vi "Rectangle1005.vi"   [LabVIEW 2013]
uses:
  <vilib>/Heliosphere Research LLC/Advanced Plotting Toolkit/api_core/NewPlotProperties.ctl
  <vilib>/Heliosphere Research LLC/Advanced Plotting Toolkit/typedefs/PlotColor.ctl
  <vilib>/Heliosphere Research LLC/Advanced Plotting Toolkit/api_annotations/ShapeProperties.ctl
  <vilib>/Heliosphere Research LLC/Advanced Plotting Toolkit/properties/Line.ctl
  <vilib>/Heliosphere Research LLC/Advanced Plotting Toolkit/properties/Line_Style.ctl
  <vilib>/Heliosphere Research LLC/Advanced Plotting Toolkit/properties/Display.ctl
  <vilib>/Heliosphere Research LLC/Advanced Plotting Toolkit/Advanced Plotting Toolkit.lvlib
types:
  T1 = typedef "Advanced Plotting Toolkit.lvlib/ShapeProperties.ctl" = cluster{"Color":T2, "Line":T3, "Display":T5}
  T2 = typedef "Advanced Plotting Toolkit.lvlib/PlotColor.ctl" = u32
  T3 = typedef "Advanced Plotting Toolkit.lvlib/Line.ctl" = cluster{"Style":T4, "Color":T2, "Width":sgl}
  T4 = typedef "Advanced Plotting Toolkit.lvlib/Line_Style.ctl" = enum16{"Automatic", "Solid", "Dashed", "Dotted", "Dash-dot", "Invisible"}
  T5 = typedef "Advanced Plotting Toolkit.lvlib/Display.ctl" = cluster{"Alpha":dbl, "Z Order":dbl}
  T6 = typedef "Advanced Plotting Toolkit.lvlib/NewPlotProperties.ctl" = cluster{"Background Color":T2, "Axis Background":T2, "Left Margin":dbl, "Right Margin":dbl, "Bottom Margin":dbl, "Top Margin":dbl, "Aspect Ratio":dbl}
  T7 = typedef "Advanced Plotting Toolkit.lvlib/PlotID.ctl" = i32
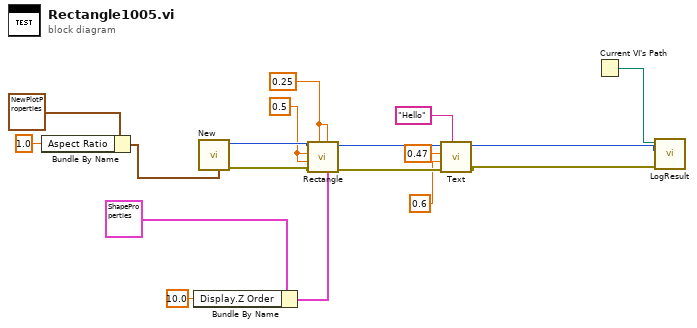
[diagram p0: block diagram]
diagram:
  w3 = 0.25 ("Radius")
  w5 = 0.5 ("X Position")
  n1 = Bundle By Name(cluster=T6 {"Background Color"=2147483647, "Axis Background"=2147483647, "Left Margin"=nan, "Right Margin"=nan, "Bottom Margin"=nan, "Top Margin"=nan, "Aspect Ratio"=nan} ("New Plot Properties"), "Aspect Ratio"=1.0) -> (w14:T6)
  n2 = Bundle By Name(cluster=T1 {"Color"=2147483647, "Line"={"Style"=enum."Automatic", "Color"=2147483647, "Width"=nan}, "Display"={"Alpha"=nan, "Z Order"=nan}} ("Shape Properties"), "Display.Z Order"=10.0 ("Display.Alpha")) -> (w11:T1)
  n3 = call <vilib>:"New.vi"("Properties"=w14) -> ("error out"=w16:errorcluster, "Plot ID"=w17:T7)  [unwired: 9 in]
  n4 = call <vilib>:"Rectangle.vi"("Properties"=w11, "Height"=w3, "Width"=w3, "error in (no error)"=w16, "Y Position"=w5, "X Position"=w5, "Plot ID"=w17) -> ("error out"=w6:errorcluster, "Plot ID Out"=w9:T7)  [unwired: 3 in]
  n5 = call <vilib>:"Text.vi"("Text"="Hello", "error in (no error)"=w6, "Y Position"=0.6, "X Position"=0.47, "Plot ID"=w9) -> ("error out"=w7:errorcluster, "Plot ID Out"=w8:T7)  [unwired: 5 in]
  n6 = Current VI's Path() -> (path=w18:path)
  n7 = call "LogResult.vi"("Test Result"=w7, "Test Artifact"=w8, "VI Path"=w18) -> ()  [unwired: 9 in]
